vi "Properties_Move Up Down Element Order.vi"(7 "Action":T2=enum."Bundler Move Up", 10 "Properties for Tree Out":T1(array[cluster]), 11 "Affected Items":T3) -> (3 "Properties for Tree Out":T1(array[cluster]))   [LabVIEW 2023]
uses:
  top/BundleMagic.ctl
  controls/action enum.ctl
panel:
  # "Using Bundler Move Up and Bundler Move Down only"
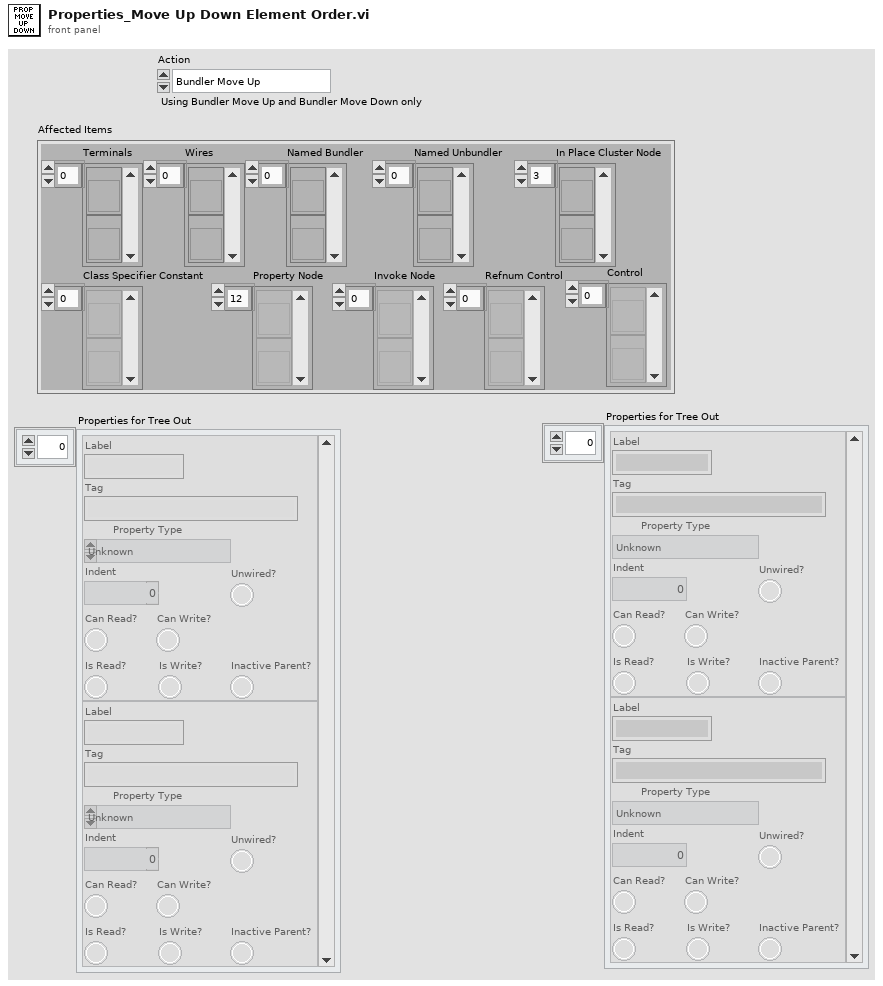
[diagram p1: front panel]
types:
  T1 = cluster{"Label":string, "Tag":string, "Property Type":enum16{"Unknown", "Base", "Scripting", "Private", "Deprecated", "None", "Divider"}, "Indent":u16, "Can Read?":bool, "Can Write?":bool, "Is Read?":bool, "Is Write?":bool, "Inactive Parent?":bool, "Unwired?":bool}[]
  T2 = typedef "action enum.ctl" = enum16{"[NONE]", "Wire Bundle", "Wire Unbundle", "Terminal Unbundle", "Terminal Bundle", "Bundler Move Up", "Bundler Move Down", "Bundler Insert", "Bundler Remove", "Bundler Remove Unwired", "Bundler Rearrange", "In Place Insert", "In Place Remove", "In Place Remove Unwired", "In Place Rearrange", "Wire Properties", "Wire Method", "Terminal Properties", "Terminal Method", "Property Move Up", "Property Move Down", "Properties Insert", "Properties Remove", "Properties Remove Unwired", "Properties Rearrange", "Method Change", "Class for Constant", "Class For Control", "Class For Node", "Class Name to Clipboard"}
  T3 = typedef "BundleMagic.ctl" = cluster{"Terminals":refnum<vi>[], "Wires":refnum<vi>[], "Named Bundler":refnum<vi>[], "Named Unbundler":refnum<vi>[], "In Place Cluster Node":refnum<vi>[], "Class Specifier Constant":refnum<vi>[], "Property Node":refnum<vi>[], "Invoke Node":refnum<vi>[], "Refnum Control":refnum<vi>[], "Control":refnum<vi>[]}
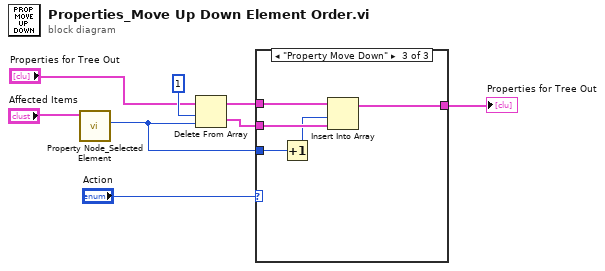
[diagram p0: block diagram]
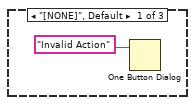
[diagram p2: hidden frame]
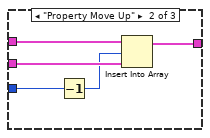
[diagram p3: hidden frame]
diagram:
  n1 = call "Property Node_Selected Element.vi"("Affected Items"="Affected Items") -> ("index of element"=w1:i32)  [unwired: 5 in, 5 out]
  n2 = Delete From Array(array="Properties for Tree Out", length=1 ("index of element"), index=w1) -> (deleted portion=w7:T1, array with subset deleted=w8:T1)
  n3 = case shown="\"Property Move Down\"" "Action" {
    tunnel: w8 -> [_ w14 w19]
    tunnel: w7 -> [_ w13 w18]
    tunnel: w1 -> [_ w12 w16]
    tunnel: [_ w10 w17] -> w5
    frame "[NONE]", Default {
      n4 = One Button Dialog(message="Invalid Action") -> ()  [unwired: 1 in, 1 out]
    }
    frame "Property Move Up" {
      n5 = Decrement(x=w12) -> (x-1=w11:i32)
      n6 = Insert Into Array(array=w14, index=w11, new element=w13) -> (w10:T1)
    }
    frame "Property Move Down" {
      n7 = Increment(x=w16) -> (x+1=w15:i32)
      n8 = Insert Into Array(array=w19, index=w15, new element=w18) -> (w17:T1)
    }
  }
  "Properties for Tree Out" <- w5
